vi "Expansion.vi"() -> ()   [LabVIEW 2014]
uses:
  <vilib>/myRIO/Instrument Drivers/Onboard IO/DIO/typedefs/DIO Reference.ctl
  <vilib>/myRIO/Common/Instrument Driver Framework/Utilities/typedefs/myRIO Generic Hardware Reference.ctl
  <vilib>/myRIO/Common/Instrument Driver Framework/Utilities/typedefs/Hardware Version Enum.ctl
  <vilib>/myRIO/Common/Instrument Driver Framework/Utilities/typedefs/myRIO v1.0 Reference.ctl
  <vilib>/myRIO/Common/Instrument Driver Framework/Utilities/typedefs/Generic FPGA Reference.ctl
  <vilib>/myRIO/Common/Instrument Driver Framework/myRIO v1.0/DIO/typedefs/DIO Channels List.ctl
  <vilib>/myRIO/Common/Instrument Driver Framework/myRIO v1.0/DIO/typedefs/DIO Channels Enum.ctl
  <vilib>/userdefined/High Color/nirio_resource_hc.ctl
  <vilib>/myRIO/Common/Instrument Driver Framework/Utilities/vis/Is FPGA Ref Available.vi
  <vilib>/myRIO/Common/Instrument Driver Framework/myRIO v1.0/DIO/vis/myRIO v1.1 Open DIO.vi
  <vilib>/myRIO/Instrument Drivers/Onboard IO/DIO/vis/Write.vi
  <vilib>/myRIO/Common/Instrument Driver Framework/Utilities/vis/Validate Channels.vi
  <vilib>/myRIO/Common/Instrument Driver Framework/myRIO v1.0/DIO/vis/myRIO v1.0 Reserve DIO.vi
  <vilib>/myRIO/Common/Instrument Driver Framework/myRIO v1.0/Resource Manager/vis/myRIO v1.0 Reserve Channel List.vi
  <vilib>/myRIO/Common/Instrument Driver Framework/myRIO v1.0/DIO/vis/myRIO v1.0 Build MUX Configuration DIO.vi
  <vilib>/myRIO/Common/Instrument Driver Framework/myRIO v1.0/Resource Manager/vis/myRIO v1.0 Reserve Channel.vi
  <vilib>/myRIO/Common/Instrument Driver Framework/myRIO v1.0/Resource Manager/vis/myRIO v1.0 Unreserve Channel.vi
  <vilib>/myRIO/Common/Instrument Driver Framework/myRIO v1.0/Resource Manager/vis/myRIO v1.0 Create Configuration List.vi
  <vilib>/myRIO/Common/Instrument Driver Framework/myRIO v1.0/Resource Manager/vis/myRIO v1.0 Build Mutex Name.vi
  <vilib>/Utility/VariantDataType/GetNumericInfo.vi
  <vilib>/Utility/error.llb/Error Cluster From Error Code.vi
  <vilib>/myRIO/Common/Instrument Driver Framework/myRIO v1.0/myRIO v1.1 Open.vi
  <vilib>/myRIO/Common/Instrument Driver Framework/Utilities/vis/IO Manager.vi
  <vilib>/myRIO/Common/Instrument Driver Framework/Utilities/vis/Configuration Manager.vi
  <vilib>/myRIO/Common/Instrument Driver Framework/myRIO v1.0/Resource Manager/vis/myRIO v1.0 Configure IO.vi
  <vilib>/myRIO/Common/Instrument Driver Framework/myRIO v1.0/myRIO v1.0 Close.vi
  <vilib>/myRIO/Common/Instrument Driver Framework/myRIO v1.0/DIO/vis/myRIO v1.0 Write DIO.vi
  <vilib>/myRIO/Express VI/Onboard IO/DO/DO Express VI.xnode
  <vilib>/myRIO/Instrument Drivers/Onboard IO/DIO/vis/myRIO DIO Open.xnode
  <vilib>/myRIO/Instrument Drivers/Onboard IO/DIO/DIO.lvlib
panel:
  in  "set time":timestamp
  out "Second Tens":bool[](array[boolean]) caption="Seconds"
  out "Second Ones":bool[](array[boolean])
  out "Minute Ones":bool[](array[boolean])
  out "Minute Tens":bool[](array[boolean]) caption="Minutes"
  in  "Stop Button":bool
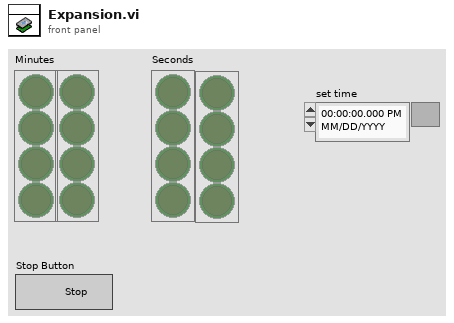
[diagram p1: front panel]
types:
  T1 = typedef "DIO.lvlib/DIO Reference.ctl" = cluster{"myRIO Reference":T2, "DIO Channels List":T6}
  T2 = typedef "myRIO Generic Hardware Reference.ctl" = cluster{"myRIO Model":T3, "myRIO Hardware Reference":T4}
  T3 = typedef "Hardware Version Enum.ctl" = enum16{"Unknown", "myRIO-1900", "myRIO-1950"}
  T4 = typedef "myRIO v1.0 Reference.ctl" = cluster{"Generic FPGA Reference":T5, "Allow multiple opens":bool}
  T5 = typedef "Generic FPGA Reference.ctl" = refnum<k20>
  T6 = typedef "DIO Channels List.ctl" = T7[]
  T7 = typedef "DIO Channels Enum.ctl" = enum16{"Not Connected", "C/DIO0", "C/DIO1", "C/DIO2", "C/DIO3", "C/DIO4", "C/DIO5", "C/DIO6", "C/DIO7", "A/DIO0", "A/DIO1", "A/DIO2", "A/DIO3", "A/DIO4", "A/DIO5", "A/DIO6", "A/DIO7", "A/DIO8", "A/DIO9", "A/DIO10", "A/DIO11", "A/DIO12", "A/DIO13", "A/DIO14", "A/DIO15", "B/DIO0", "B/DIO1", "B/DIO2", "B/DIO3", "B/DIO4", "B/DIO5", "B/DIO6", "B/DIO7", "B/DIO8", "B/DIO9", "B/DIO10", "B/DIO11", "B/DIO12", "B/DIO13", "B/DIO14", "B/DIO15", "LED0", "LED1", "LED2", "LED3", "Button0"}
  T8 = typedef "nirio_resource_hc.ctl" = tag
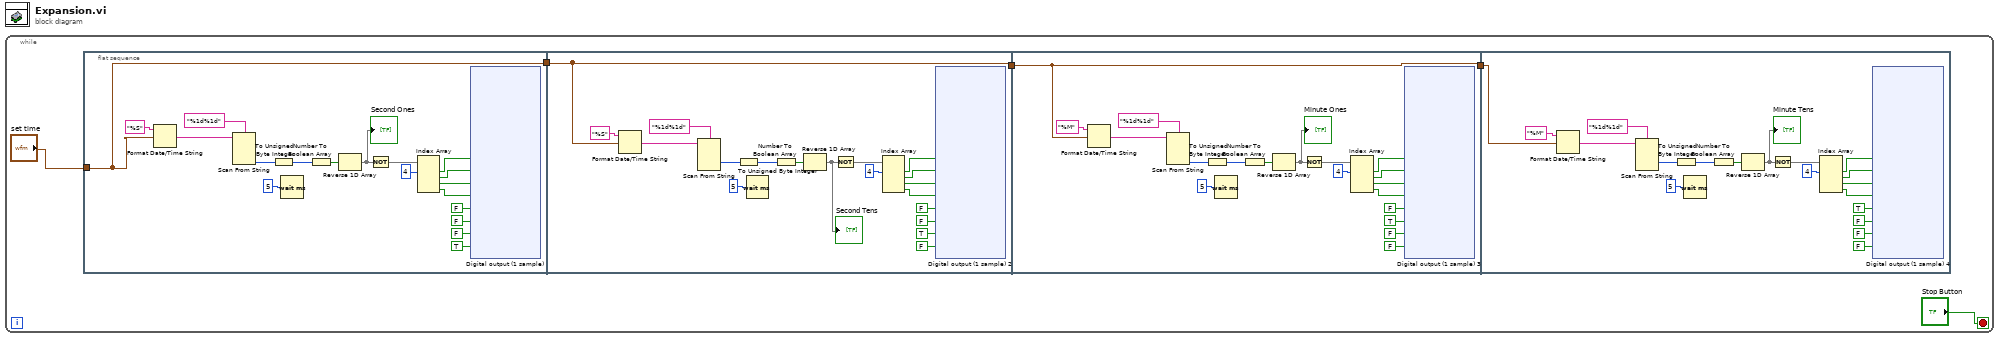
[diagram p0: block diagram]
diagram:
  n1 = while {
    stop <- "Stop Button" stop-if-true
    n2 = flat-sequence {
      tunnel: "set time" -> [w6]
      tunnel: [w6] -> w3
      tunnel: w3 -> [w67]
      tunnel: [w67] -> w2
      tunnel: w2 -> [w128]
      tunnel: [w128] -> w1
      tunnel: w1 -> [w189]
      frame #0 {
        n3 = Format Date/Time String(time format string (%c)="%S", seconds (now)=w6) -> (date/time string=w22:string)  [unwired: 1 in]
        n4 = Scan From String(format string="%1d%1d", input string=w22) -> (output 2=w20:i32)  [unwired: 5 in, 3 out]
        n5 = To Unsigned Byte Integer(number=w20) -> (unsigned 8bit integer=w21:u8)
        n6 = Wait (ms)(milliseconds to wait=u32 5) -> ()  [unwired: 1 out]
        n7 = Number To Boolean Array(number=w21) -> (Boolean array=w10:bool[])
        n8 = Reverse 1D Array(array=w10) -> (reversed array=w8:bool[])
        "Second Ones" <- w8
        n9 = Not(x=w8) -> (.not. x?=w9:bool[])
        n10 = Index Array(array=w9, index #1=4 ("index")) -> (element #1=w14:bool, element #2=w13:bool, element #3=w12:bool, element #4=w11:bool)  [unwired: 3 in]
        n11 = xnode "Digital output (1 sample)"("B/DIO0 (Pin 11)"=w14, "B/DIO1 (Pin 13)"=w13, "B/DIO2 (Pin 15)"=w12, "B/DIO3 (Pin 17)"=w11, "B/DIO4 (Pin 19)"=FALSE ("B/DIO7 (Pin 25)"), "B/DIO5 (Pin 21)"=FALSE ("B/DIO7 (Pin 25)"), "B/DIO6 (Pin 23)"=FALSE ("B/DIO7 (Pin 25)"), "B/DIO7 (Pin 25)"=TRUE) -> ()  [unwired: 1 in, 1 out]
      }
      frame #1 {
        n12 = Format Date/Time String(time format string (%c)="%S", seconds (now)=w67) -> (date/time string=w85:string)  [unwired: 1 in]
        n13 = Scan From String(format string="%1d%1d", input string=w85) -> (output 1=w83:i32)  [unwired: 5 in, 3 out]
        n14 = To Unsigned Byte Integer(number=w83) -> (unsigned 8bit integer=w82:u8)
        n15 = Wait (ms)(milliseconds to wait=u32 5) -> ()  [unwired: 1 out]
        n16 = Number To Boolean Array(number=w82) -> (Boolean array=w71:bool[])
        n17 = Reverse 1D Array(array=w71) -> (reversed array=w70:bool[])
        "Second Tens" <- w70
        n18 = Not(x=w70) -> (.not. x?=w69:bool[])
        n19 = Index Array(array=w69, index #1=4 ("index")) -> (element #1=w75:bool, element #2=w74:bool, element #3=w73:bool, element #4=w72:bool)  [unwired: 3 in]
        n20 = xnode "Digital output (1 sample) 2"("B/DIO0 (Pin 11)"=w75, "B/DIO1 (Pin 13)"=w74, "B/DIO2 (Pin 15)"=w73, "B/DIO3 (Pin 17)"=w72, "B/DIO4 (Pin 19)"=FALSE ("B/DIO7 (Pin 25)"), "B/DIO5 (Pin 21)"=FALSE ("B/DIO7 (Pin 25)"), "B/DIO6 (Pin 23)"=TRUE ("B/DIO7 (Pin 25)"), "B/DIO7 (Pin 25)"=FALSE) -> ()  [unwired: 1 in, 1 out]
      }
      frame #2 {
        n21 = Format Date/Time String(time format string (%c)="%M", seconds (now)=w128) -> (date/time string=w144:string)  [unwired: 1 in]
        n22 = Scan From String(format string="%1d%1d", input string=w144) -> (output 2=w141:i32)  [unwired: 5 in, 3 out]
        n23 = To Unsigned Byte Integer(number=w141) -> (unsigned 8bit integer=w143:u8)
        n24 = Wait (ms)(milliseconds to wait=u32 5) -> ()  [unwired: 1 out]
        n25 = Number To Boolean Array(number=w143) -> (Boolean array=w142:bool[])
        n26 = Reverse 1D Array(array=w142) -> (reversed array=w129:bool[])
        "Minute Ones" <- w129
        n27 = Not(x=w129) -> (.not. x?=w131:bool[])
        n28 = Index Array(array=w131, index #1=4 ("index")) -> (element #1=w135:bool, element #2=w134:bool, element #3=w133:bool, element #4=w132:bool)  [unwired: 3 in]
        n29 = xnode "Digital output (1 sample) 3"("B/DIO0 (Pin 11)"=w135, "B/DIO1 (Pin 13)"=w134, "B/DIO2 (Pin 15)"=w133, "B/DIO3 (Pin 17)"=w132, "B/DIO4 (Pin 19)"=FALSE ("B/DIO7 (Pin 25)"), "B/DIO5 (Pin 21)"=TRUE ("B/DIO7 (Pin 25)"), "B/DIO6 (Pin 23)"=FALSE ("B/DIO7 (Pin 25)"), "B/DIO7 (Pin 25)"=FALSE) -> ()  [unwired: 1 in, 1 out]
      }
      frame #3 {
        n30 = Format Date/Time String(time format string (%c)="%M", seconds (now)=w189) -> (date/time string=w207:string)  [unwired: 1 in]
        n31 = Scan From String(format string="%1d%1d", input string=w207) -> (output 1=w203:i32)  [unwired: 5 in, 3 out]
        n32 = To Unsigned Byte Integer(number=w203) -> (unsigned 8bit integer=w204:u8)
        n33 = Wait (ms)(milliseconds to wait=u32 5) -> ()  [unwired: 1 out]
        n34 = Number To Boolean Array(number=w204) -> (Boolean array=w202:bool[])
        n35 = Reverse 1D Array(array=w202) -> (reversed array=w190:bool[])
        "Minute Tens" <- w190
        n36 = Not(x=w190) -> (.not. x?=w192:bool[])
        n37 = Index Array(array=w192, index #1=4 ("index")) -> (element #1=w196:bool, element #2=w195:bool, element #3=w194:bool, element #4=w193:bool)  [unwired: 3 in]
        n38 = xnode "Digital output (1 sample) 4"("B/DIO0 (Pin 11)"=w196, "B/DIO1 (Pin 13)"=w195, "B/DIO2 (Pin 15)"=w194, "B/DIO3 (Pin 17)"=w193, "B/DIO4 (Pin 19)"=TRUE ("B/DIO7 (Pin 25)"), "B/DIO5 (Pin 21)"=FALSE ("B/DIO7 (Pin 25)"), "B/DIO6 (Pin 23)"=FALSE ("B/DIO7 (Pin 25)"), "B/DIO7 (Pin 25)"=FALSE) -> ()  [unwired: 1 in, 1 out]
      }
    }
  }
